vi "test11.vi"() -> ()   [LabVIEW 2010]
panel:
  in  "gamma2":dbl=1.0
  in  "omega2":dbl=5.0
  in  "gamm1":dbl=0.05
  in  "omega1":dbl=1.0
  in  "factor":dbl=3.0
  out "real axis":dbl[](array[numeric])=[-0.001573233, -0.0015680711305333334, -0.0015629092610666667, -0.0015577473916, -0.0015525855221333333, -0.0015474236526666666, -0.0015422617832000001, -0.0015370999137333335, -0.0015319380442666668, -0.0015267761748, -0.0015216143053333334, -0.0015164524358666667, -0.0015112905664, -0.0015061286969333333, -0.0015009668274666666, -0.001495804958, -0.0014906430885333333, -0.0014854812190666668, -0.0014803193496000001, -0.0014751574801333334, -0.0014699956106666667, -0.0014648337412, -0.0014596718717333334, -0.0014545100022666667, -0.0014493481328, -0.0014441862633333333, -0.0014390243938666668, -0.0014338625244000001, -0.0014287006549333335, -0.0014235387854666668, -0.001418376916, -0.0014132150465333334, -0.0014080531770666667, -0.0014028913076, -0.0013977294381333333, -0.0013925675686666666, -0.0013874056992, -0.0013822438297333333, -0.0013770819602666666, -0.0013719200908000001, -0.0013667582213333334, -0.0013615963518666667, -0.0013564344824, -0.0013512726129333334, -0.0013461107434666667, -0.001340948874, -0.0013357870045333333, -0.0013306251350666666, -0.0013254632656000001, -0.0013203013961333335, -0.0013151395266666668, -0.0013099776572, -0.0013048157877333334, -0.0012996539182666667, -0.0012944920488, -0.0012893301793333333, -0.0012841683098666666, -0.0012790064404, -0.0012738445709333333, -0.0012686827014666666, -0.001263520832, -0.0012583589625333334, -0.0012531970930666667, -0.0012480352236, -0.0012428733541333334, -0.0012377114846666667, -0.0012325496152, -0.0012273877457333333, -0.0012222258762666668, -0.0012170640068000001, -0.0012119021373333335, -0.0012067402678666668, -0.0012015783984, -0.0011964165289333334, -0.0011912546594666667, -0.00118609279, -0.0011809309205333333, -0.0011757690510666666, -0.0011706071816, -0.0011654453121333333, -0.0011602834426666666, -0.0011551215731999999, -0.0011499597037333334, -0.0011447978342666667, -0.0011396359648, -0.0011344740953333334, -0.0011293122258666667, -0.0011241503564, -0.0011189884869333333, -0.0011138266174666666, -0.0011086647480000001, -0.0011035028785333334, -0.0010983410090666668, -0.0010931791396, -0.0010880172701333334, -0.0010828554006666667, -0.0010776935312, -0.0010725316617333333, -0.0010673697922666666, -0.0010622079228, -0.0010570460533333333, -0.0010518841838666666, -0.0010467223143999999, -0.0010415604449333332, -0.0010363985754666667, -0.001031236706, -0.0010260748365333334, -0.0010209129670666667, -0.0010157510976, -0.0010105892281333333, -0.0010054273586666668, -0.0010002654892000001, -0.0009951036197333334, -0.0009899417502666668, -0.0009847798808, -0.0009796180113333334, -0.0009744561418666667, -0.0009692942724, -0.0009641324029333333, -0.0009589705334666666, -0.000953808664, -0.0009486467945333334, -0.0009434849250666667, -0.0009383230556, -0.0009331611861333333, -0.0009279993166666666, -0.0009228374472, -0.0009176755777333334, -0.0009125137082666667, -0.0009073518388, -0.0009021899693333333, -0.0008970280998666667, -0.0008918662304, -0.0008867043609333333, -0.0008815424914666666, -0.000876380622, -0.0008712187525333334, -0.0008660568830666667, -0.0008608950136, -0.0008557331441333333, -0.0008505712746666666, -0.0008454094052, -0.0008402475357333334, -0.0008350856662666667, -0.0008299237968, -0.0008247619273333333, -0.0008196000578666666, -0.0008144381884, -0.0008092763189333334, -0.0008041144494666667, -0.00079895258, -0.0007937907105333333, -0.0007886288410666666, -0.0007834669716, -0.0007783051021333333, -0.0007731432326666666, -0.0007679813632, -0.0007628194937333333, -0.0007576576242666667, -0.0007524957548, -0.0007473338853333333, -0.0007421720158666666, -0.0007370101463999999, -0.0007318482769333334, -0.0007266864074666667, -0.000721524538, -0.0007163626685333333, -0.0007112007990666666, -0.0007060389296, -0.0007008770601333333, -0.0006957151906666667, -0.0006905533212, -0.0006853914517333333, -0.0006802295822666666, -0.0006750677128, -0.0006699058433333333, -0.0006647439738666666, -0.0006595821044, -0.0006544202349333333, -0.0006492583654666667, -0.000644096496, -0.0006389346265333333, -0.0006337727570666666, -0.0006286108875999999, -0.0006234490181333333, -0.0006182871486666667, -0.0006131252792, -0.0006079634097333333, -0.0006028015402666666, -0.0005976396707999999, -0.0005924778013333333, -0.0005873159318666667, -0.0005821540624, -0.0005769921929333333, -0.0005718303234666666, -0.0005666684539999999, -0.0005615065845333332, -0.0005563447150666665, -0.0005511828456000001, -0.0005460209761333334, -0.0005408591066666667, -0.0005356972372, -0.0005305353677333333, -0.0005253734982666666, -0.0005202116287999999, -0.0005150497593333333, -0.0005098878898666666, -0.0005047260203999999, -0.0004995641509333334, -0.0004944022814666667, -0.000489240412, -0.00048407854253333335, -0.00047891667306666666, -0.00047375480359999997, -0.0004685929341333333, -0.0004634310646666666, -0.0004582691951999999, -0.0004531073257333332, -0.00044794545626666653, -0.00044278358680000006, -0.0004376217173333334, -0.0004324598478666667, -0.0004272979784, -0.0004221361089333333, -0.0004169742394666666, -0.00041181236999999994, -0.00040665050053333325, -0.00040148863106666656, -0.0003963267615999999, -0.0003911648921333332, -0.0003860030226666667, -0.00038084115320000003, -0.00037567928373333334, -0.00037051741426666666, -0.00036535554479999997, -0.0003601936753333333, -0.0003550318058666666, -0.0003498699363999999, -0.0003447080669333332, -0.00033954619746666653, -0.00033438432799999984, -0.0003292224585333334, -0.0003240605890666667, -0.0003188987196, -0.0003137368501333333, -0.0003085749806666666, -0.00030341311119999994, -0.00029825124173333325, -0.00029308937226666656, -0.0002879275027999999, -0.0002827656333333332, -0.0002776037638666667, -0.00027244189440000003, -0.00026728002493333334, -0.00026211815546666665, -0.00025695628599999997, -0.0002517944165333333, -0.0002466325470666666, -0.0002414706775999999, -0.00023630880813333322, -0.00023114693866666653, -0.00022598506919999984, -0.00022082319973333337, -0.00021566133026666668, -0.0002104994608, -0.0002053375913333333, -0.00020017572186666662, -0.00019501385239999993, -0.00018985198293333325, -0.00018469011346666656, -0.00017952824399999987, -0.00017436637453333318, -0.00016920450506666671, -0.00016404263560000003, -0.00015888076613333334, -0.00015371889666666665, -0.00014855702719999996, -0.00014339515773333328, -0.0001382332882666666, -0.0001330714187999999, -0.00012790954933333321, -0.00012274767986666653, -0.00011758581039999984, -0.00011242394093333337, -0.00010726207146666668, -0.000102100202, -9.69383325333333e-05, -9.177646306666662e-05, -8.661459359999993e-05, -8.145272413333324e-05, -7.629085466666656e-05, -7.112898519999987e-05, -6.596711573333318e-05, -6.0805246266666495e-05, -5.5643376800000024e-05, -5.048150733333334e-05, -4.531963786666665e-05, -4.015776839999996e-05, -3.4995898933333274e-05, -2.9834029466666587e-05]
  out "Array":cdb[](array[numeric])
  in  "center gamma":dbl=2.0
  in  "delta gamma":dbl=3.9
  in  "dimension size br cut":i32=500
  in  "center omega":dbl
  in  "delta omega":dbl=10.0
  in  "omega range":dbl=500.0
  in  "dimension size":i32=5000
  out "Plot: frequency vs T":cluster{dbl[], dbl[]}[](graph)
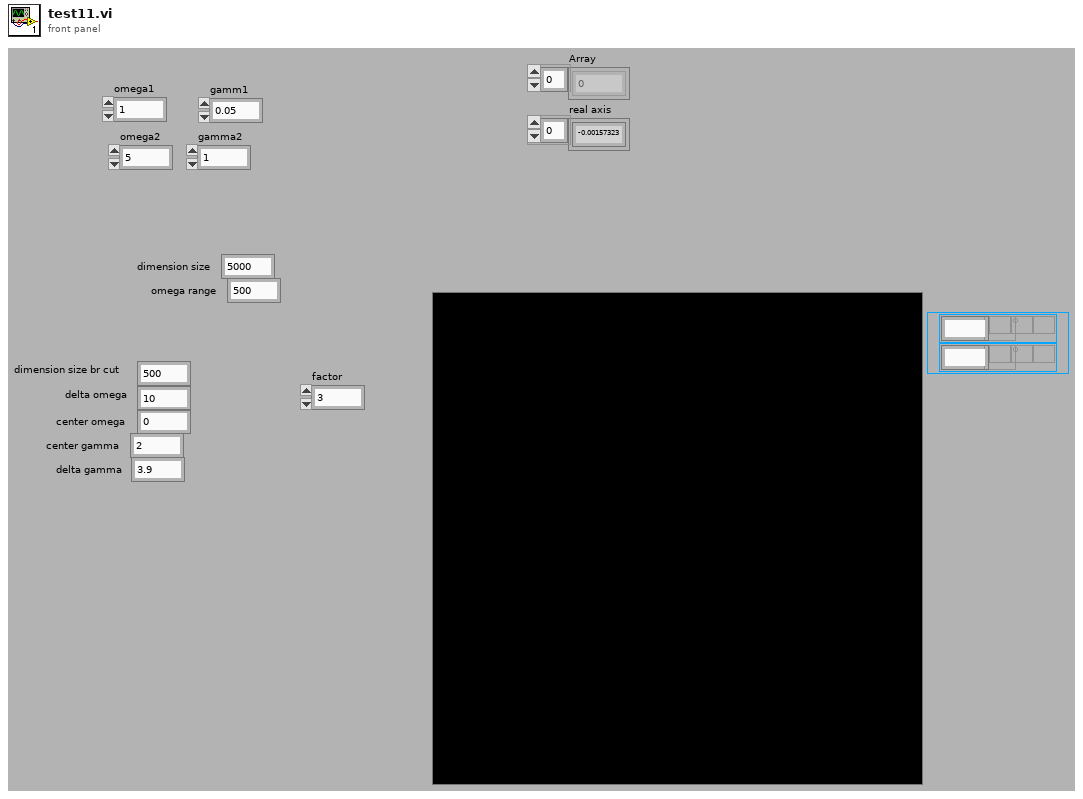
[diagram p1: front panel]
types:
  T1 = typedef "LVCursorListTypeDef.ctl" = cluster{"Name":string, "Color":u32, "Style":u8, "Point Style":u8, "Name Visible":bool, "Allow Drag":bool, "Cursor Mode":u32, "Plot":i32, "Index":i32, "Position":cluster{"X":dbl, "Y":dbl}, "X Scale":u32, "Y Scale":u32, "Watch Plots":i32[], "Watch All Plots":bool, "Plot Area":i32, "Label Offset":cluster{"X":dbl, "Y":dbl}}[]
  T2 = cluster{"Name":string, "Color":u32, "Style":u8, "Point Style":u8, "Name Visible":bool, "Allow Drag":bool, "Cursor Mode":u32, "Plot":i32, "Index":i32, "Position":cluster{"X":dbl, "Y":dbl}, "X Scale":u32, "Y Scale":u32, "Watch Plots":i32[], "Watch All Plots":bool, "Plot Area":i32, "Label Offset":cluster{"X":dbl, "Y":dbl}}
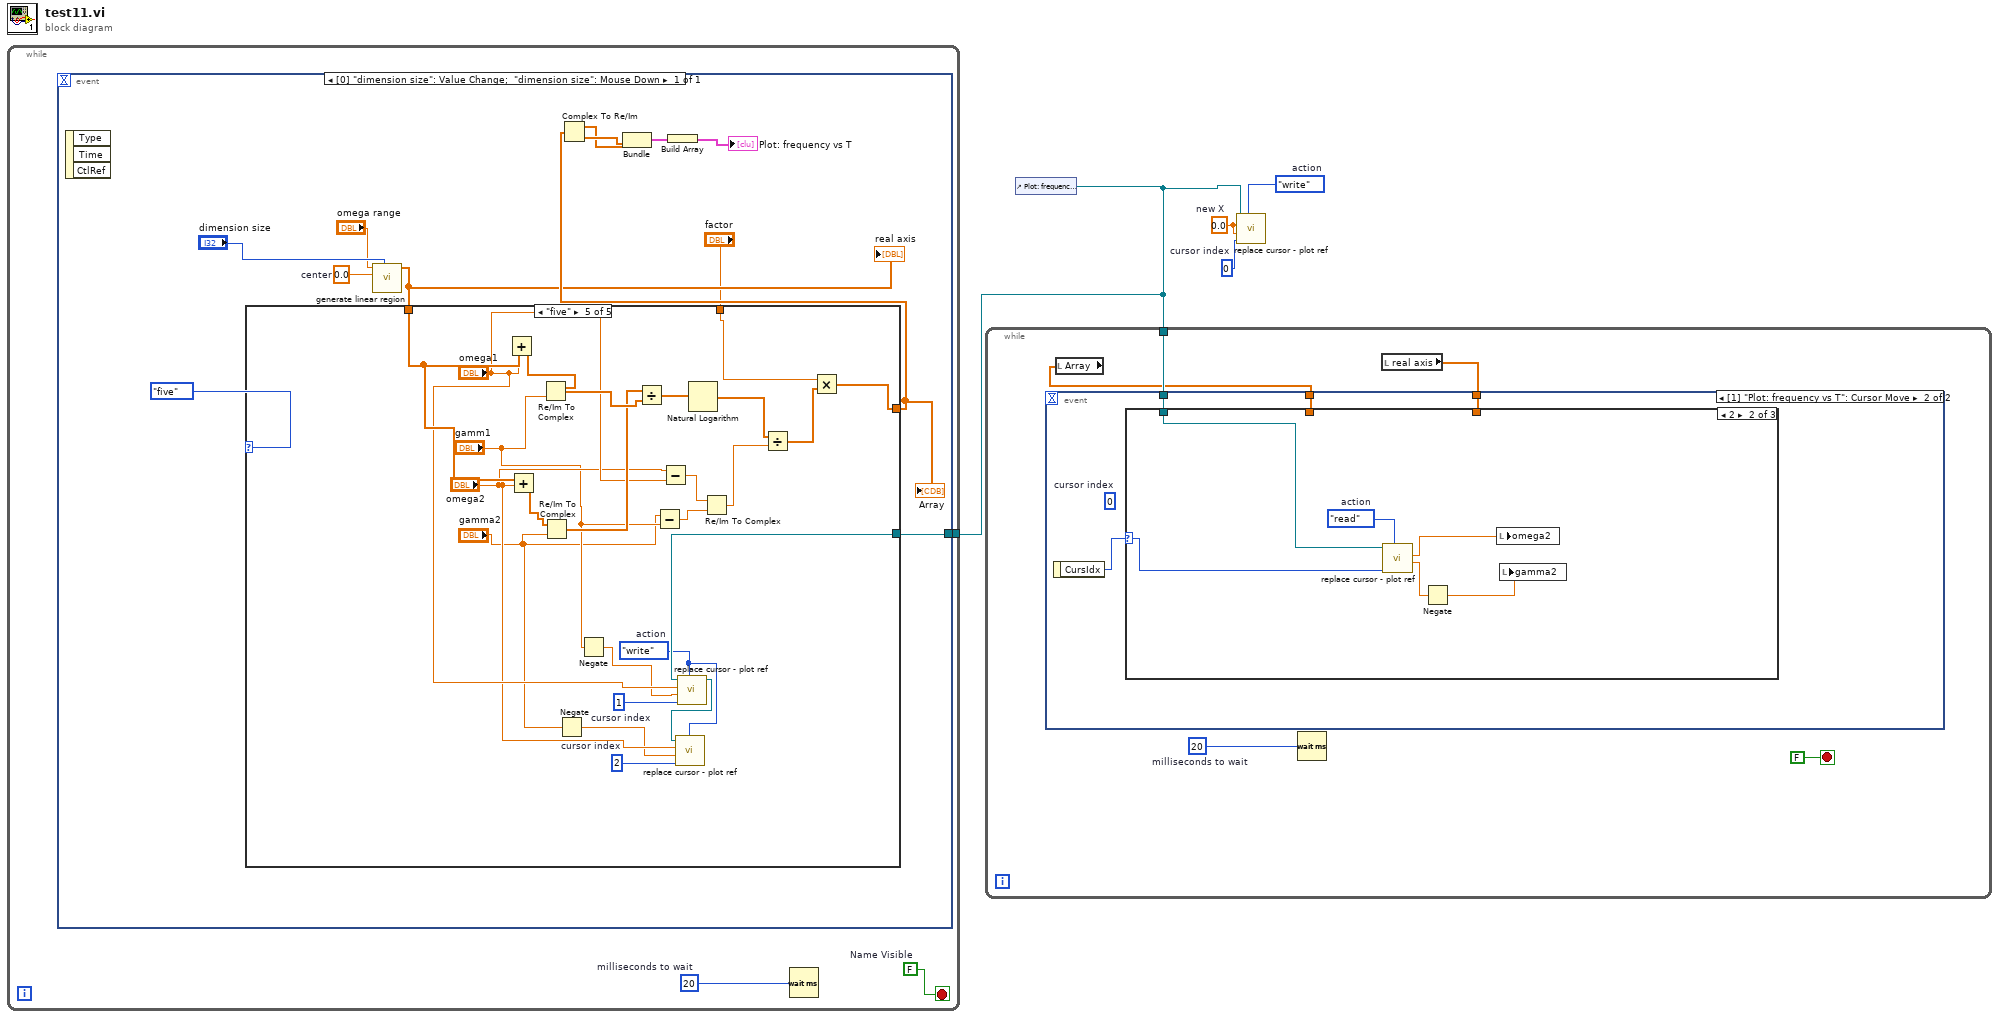
[diagram p0: block diagram]
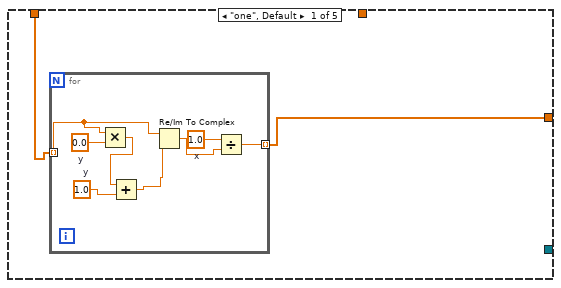
[diagram p2: hidden frame]
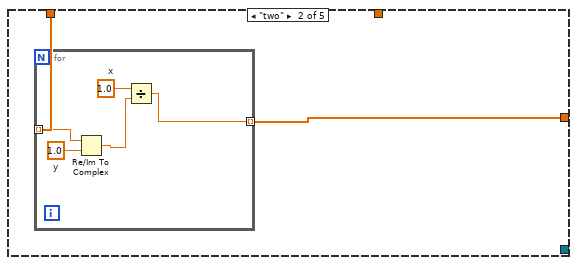
[diagram p3: hidden frame]
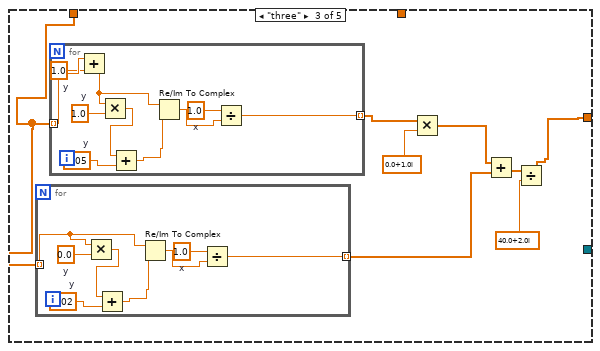
[diagram p4: hidden frame]
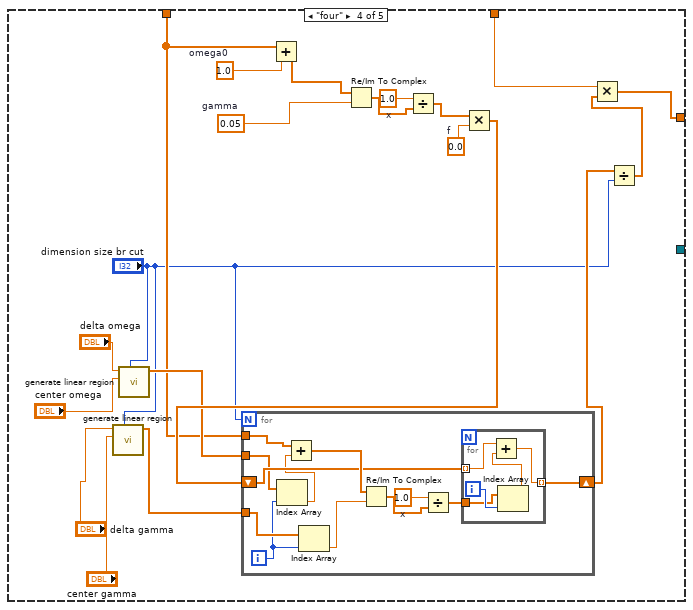
[diagram p5: hidden frame]
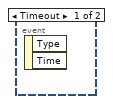
[diagram p6: hidden frame]
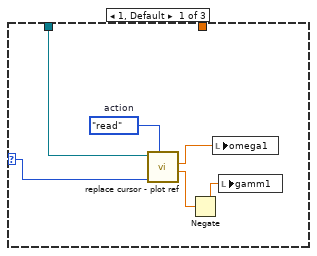
[diagram p7: hidden frame]
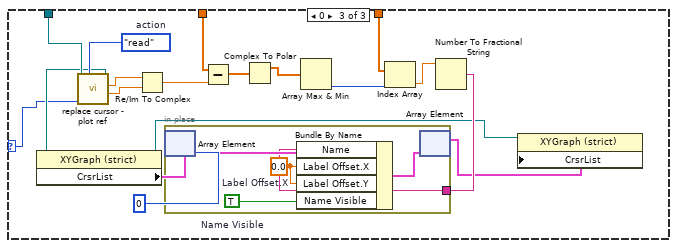
[diagram p8: hidden frame]
diagram:
  w2 = 0.0  # new X
  w3 = enum16{"", "read", "write"}."write"  # action
  w4 = 0  # cursor index
  n1 = control-ref of="Plot: frequency vs T"() -> (w1:refnum<vi>)
  n2 = while {
    tunnel: w1 -> [w5]
    stop <- w6 stop-if-true
    w6 = FALSE  # Name Visible
    w7 = u32 20  # milliseconds to wait
    n3 = event shown="[0] \"dimension size\": Value Change;  \"dimension size\": Mouse Down" {
      selector: _ -> [_]
      dyn-events: _ -> [_]
      timeout: _ -> [_]
      tunnel: w5 -> [w8]
      event "dimension size": Value Change; "dimension size": Mouse Down {
        w15 = 0.0  # center
        n4 = event-data() -> ()  [unwired: 1 in, 3 out]
        n5 = call "generate linear region.vi"("number of  grid points"="dimension size", "center"=w15, "delta"="omega range") -> ("real axis"=w10:dbl[])  [unwired: 8 in]
        "real axis" <- w10
        n6 = case shown="\"five\"" enum16{"one", "three", "four", "five", "two"}."five" {
          tunnel: w10 -> [w21 w31 w44 w67 w121]
          tunnel: [w20 w30 w37 w65 w117] -> w11
          tunnel: "factor" -> [_ _ _ w63 w116]
          tunnel: w8 -> [_ _ _ _ w110]
          frame "one", Default {
            n7 = for {
              tunnel: w21 -> [w25] mode=indexing
              tunnel: [w27] -> w20 mode=indexing
              w24 = 0.0  # y
              w26 = 1.0  # y
              w29 = 1.0  # x
              n8 = Multiply(x=w25, y=w24) -> (x*y=w23:dbl)
              n9 = Add(x=w23, y=w26) -> (x+y=w22:dbl)
              n10 = Re/Im To Complex(1:w22, 2:w25) -> (0:w28:cdb)
              n11 = Divide(x=w29, y=w28) -> (x/y=w27:cdb)
            }
          }
          frame "two" {
            n12 = for {
              tunnel: w31 -> [w35] mode=indexing
              tunnel: [w32] -> w30 mode=indexing
              w34 = 1.0  # y
              w36 = 1.0  # x
              n13 = Re/Im To Complex(1:w34, 2:w35) -> (0:w33:cdb)
              n14 = Divide(x=w36, y=w33) -> (x/y=w32:cdb)
            }
          }
          frame "three" {
            n15 = for {
              tunnel: w44 -> [w48] mode=indexing
              tunnel: [w50] -> w40 mode=indexing
              w47 = 0.0  # y
              w49 = 0.02  # y
              w52 = 1.0  # x
              n16 = Multiply(x=w48, y=w47) -> (x*y=w46:dbl)
              n17 = Add(x=w46, y=w49) -> (x+y=w45:dbl)
              n18 = Re/Im To Complex(1:w45, 2:w48) -> (0:w51:cdb)
              n19 = Divide(x=w52, y=w51) -> (x/y=w50:cdb)
            }
            n20 = for {
              tunnel: w44 -> [w55] mode=indexing
              tunnel: [w60] -> w43 mode=indexing
              w54 = 1.0  # y
              w58 = 1.0  # y
              w59 = 0.05  # y
              w62 = 1.0  # x
              n21 = Add(x=w55, y=w54) -> (x+y=w53:dbl)
              n22 = Multiply(x=w53, y=w58) -> (x*y=w57:dbl)
              n23 = Add(x=w57, y=w59) -> (x+y=w56:dbl)
              n24 = Re/Im To Complex(1:w56, 2:w53) -> (0:w61:cdb)
              n25 = Divide(x=w62, y=w61) -> (x/y=w60:cdb)
            }
            n26 = Multiply(x=w43, y=cdb 0.0+1.0i) -> (x*y=w41:cdb[])
            n27 = Add(x=w41, y=w40) -> (x+y=w39:cdb[])
            n28 = Divide(x=w39, y=cdb 40.0+2.0i) -> (x/y=w37:cdb[])
          }
          frame "four" {
            w76 = 0.0  # f
            w80 = 1.0  # omega0
            w78 = 0.05  # gamma
            w82 = 1.0  # x
            n29 = call "generate linear region.vi"("number of  grid points"="dimension size br cut", "center"="center gamma", "delta"="delta gamma") -> ("real axis"=w70:dbl[])  [unwired: 8 in]
            n30 = call "generate linear region.vi"("number of  grid points"="dimension size br cut", "center"="center omega", "delta"="delta omega") -> ("real axis"=w71:dbl[])  [unwired: 8 in]
            n31 = Add(x=w67, y=w80) -> (x+y=w79:dbl[])
            n32 = Re/Im To Complex(1:w78, 2:w79) -> (0:w81:cdb[])
            n33 = Divide(x=w82, y=w81) -> (x/y=w77:cdb[])
            n34 = Multiply(x=w77, y=w76) -> (x*y=w75:cdb[])
            n35 = for {
              N: "dimension size br cut" -> [_]
              shift-right: [w88] -> w74
              shift-left: w75 -> [w90]
              tunnel: w71 -> [w83]
              tunnel: w70 -> [w87]
              tunnel: w67 -> [w92]
              i -> [w85]
              w94 = 1.0  # x
              n36 = Index Array(array=w83, index=w85) -> (element=w84:dbl)
              n37 = Add(x=w92, y=w84) -> (x+y=w93:dbl[])
              n38 = Index Array(array=w87, index=w85) -> (element=w86:dbl)
              n39 = Re/Im To Complex(1:w86, 2:w93) -> (0:w91:cdb[])
              n40 = Divide(x=w94, y=w91) -> (x/y=w89:cdb[])
              n41 = for {
                tunnel: w90 -> [w99] mode=indexing
                tunnel: w89 -> [w96]
                tunnel: [w98] -> w88 mode=indexing
                i -> [w97]
                n42 = Index Array(array=w96, index=w97) -> (element=w95:cdb)
                n43 = Add(x=w99, y=w95) -> (x+y=w98:cdb)
              }
            }
            n44 = Divide(x=w74, y="dimension size br cut") -> (x/y=w66:cdb[])
            n45 = Multiply(x=w63, y=w66) -> (x*y=w65:cdb[])
          }
          frame "five" {
            w104 = enum16{"", "read", "write"}."write"  # action
            w105 = 2  # cursor index
            w106 = 1  # cursor index
            n46 = Add(x=w121, y="omega1") -> (x+y=w122:dbl[])
            n47 = Add(x=w121, y="omega2") -> (x+y=w120:dbl[])
            n48 = Re/Im To Complex(1:"gamm1", 2:w122) -> (0:w123:cdb[])
            n49 = Re/Im To Complex(1:"gamma2", 2:w120) -> (0:w119:cdb[])
            n50 = Negate(x="gamma2") -> (-x=w100:dbl)
            n51 = Negate(x="gamm1") -> (-x=w102:dbl)
            n52 = Divide(x=w119, y=w123) -> (x/y=w118:cdb[])
            n53 = Subtract(x="gamma2", y="gamm1") -> (x-y=w115:dbl)
            n54 = Subtract(x="omega2", y="omega1") -> (x-y=w114:dbl)
            n55 = call "replace cursor - plot ref.vi"("action"=w104, "cursor index"=w106, "new  Y"=w102, "new X"="omega1", "Plot ref in"=w110) -> ("Plot ref out"=w109:refnum<vi>)  [unwired: 4 in, 2 out]
            n56 = call "replace cursor - plot ref.vi"("action"=w104, "cursor index"=w105, "new  Y"=w100, "new X"="omega2", "Plot ref in"=w109) -> ()  [unwired: 4 in, 3 out]
            n57 = Natural Logarithm(1:w118) -> (0:w113:cdb[])
            n58 = Re/Im To Complex(1:w115, 2:w114) -> (0:w112:cdb)
            n59 = Divide(x=w113, y=w112) -> (x/y=w111:cdb[])
            n60 = Multiply(x=w116, y=w111) -> (x*y=w117:cdb[])
          }
        }
        "Array" <- w11
        n61 = Complex To Re/Im(x + iy=w11) -> (x=w13:dbl[], y=w14:dbl[])
        n62 = Bundle(w13, w14) -> (w19:cluster{dbl[], dbl[]})  [unwired: 1 in]
        n63 = Build Array(w19) -> (→"Plot: frequency vs T":cluster{dbl[], dbl[]}[])
      }
    }
    n64 = Wait (ms)(milliseconds to wait=w7) -> ()  [unwired: 1 out]
  }
  n65 = while {
    tunnel: w1 -> [w126]
    stop <- FALSE stop-if-true
    w128 = u32 20  # milliseconds to wait
    n66 = local read "Array"() -> (w125:cdb[])
    n67 = Wait (ms)(milliseconds to wait=w128) -> ()  [unwired: 1 out]
    n68 = local read "real axis"() -> (w124:dbl[])
    n69 = event shown="[1] \"Plot: frequency vs T\": Cursor Move" {
      selector: _ -> [_ _]
      dyn-events: _ -> [_ _]
      timeout: _ -> [_ _]
      tunnel: w125 -> [_ w132]
      tunnel: w124 -> [_ w131]
      tunnel: w126 -> [_ w130]
      event Timeout {
        n70 = event-data() -> ()  [unwired: 1 in, 2 out]
      }
      event "Plot: frequency vs T": Cursor Move {
        (unwired) 0  # cursor index
        n71 = event-data() -> ("CursIdx"=w129:i32)  [unwired: 1 in]
        n72 = case shown="2" w129 {
          selector: w129 -> [w138 w141 w145]
          tunnel: w132 -> [_ _ w159]
          tunnel: w131 -> [_ _ w156]
          tunnel: w130 -> [w136 w142 w148]
          frame 1, Default {
            w137 = enum16{"", "read", "write"}."read"  # action
            n73 = call "replace cursor - plot ref.vi"("action"=w137, "cursor index"=w138, "Plot ref in"=w136) -> ("read Y"=w134:dbl, "read X"=w135:dbl)  [unwired: 6 in, 1 out]
            n74 = Negate(x=w134) -> (-x=w133:dbl)
            n75 = local write "omega1"(w135) -> ()
            n76 = local write "gamm1"(w133) -> ()
          }
          frame 2 {
            w144 = enum16{"", "read", "write"}."read"  # action
            n77 = call "replace cursor - plot ref.vi"("action"=w144, "cursor index"=w141, "Plot ref in"=w142) -> ("read Y"=w143:dbl, "read X"=w140:dbl)  [unwired: 6 in, 1 out]
            n78 = Negate(x=w143) -> (-x=w139:dbl)
            n79 = local write "omega2"(w140) -> ()
            n80 = local write "gamma2"(w139) -> ()
          }
          frame 0 {
            w149 = enum16{"", "read", "write"}."read"  # action
            n81 = call "replace cursor - plot ref.vi"("action"=w149, "cursor index"=w145, "Plot ref in"=w148) -> ("read Y"=w161:dbl, "read X"=w162:dbl, "Plot ref out"=w147:refnum<vi>)  [unwired: 6 in]
            n82 = property on="Property Node" class="XYGraph (strict)"(reference=w147) -> (reference out=w152:refnum<vi>, "CrsrList"=w155:T1)  [unwired: 1 in, 1 out]
            n83 = Re/Im To Complex(1:w161, 2:w162) -> (0:w160:cdb)
            n84 = Subtract(x=w159, y=w160) -> (x-y=w158:cdb[])
            n85 = Complex To Polar(r * e^(i*theta)=w158) -> (r=w146:dbl[])  [unwired: 1 out]
            n86 = Array Max & Min(array=w146) -> (min index (indices)=w157:i32)  [unwired: 3 out]
            n87 = Index Array(array=w156, index=w157) -> (element=w150:dbl)
            n88 = Number To Fractional String(number=w150) -> (F-format string=w153:string)  [unwired: 3 in]
            n89 = in-place {
              in-place-border: w153 -> [w166]
              w163 = TRUE  # Name Visible
              w164 = 0.0  # Label Offset.X
              n90 = in-place-array #1(w155, 0) -> (w167:T2)
              n91 = Bundle By Name(cluster=w167, "Name"=w166, "Label Offset.X"=w164, "Label Offset.Y"=w164, "Name Visible"=w163) -> (w165:T2)
              n92 = in-place-array #1(w165) -> (w151:T1)  [unwired: 1 out]
            }
            n93 = property on="Property Node" class="XYGraph (strict)"(reference=w152, "CrsrList"=w151) -> ()  [unwired: 1 in, 2 out]
          }
        }
      }
    }
  }
  n94 = call "replace cursor - plot ref.vi"("action"=w3, "cursor index"=w4, "new  Y"=w2, "new X"=w2, "Plot ref in"=w1) -> ()  [unwired: 4 in, 3 out]
